vi "Calculate Tip offset.vi"() -> ()   [LabVIEW 2016]
uses:
  <vilib>/Utility/file.llb/Write Delimited Spreadsheet (DBL).vi
  Classes/Controller/Motion/Motion.lvclass
  Classes/Controller/Controller.lvclass
panel:
  in  "stop":bool
  out "XYZTheta Out":dbl[](array[numeric])
  in  "Tab Control":enum32{"Page 1", "Page 2"}(tab)
  in  "Joystick P1,P2":bool
  out "Tip Offset (XY=P1-P2)":dbl[](array[numeric]) format="%#_8g"
  in  "Write Tip Offset":bool
  out "Tip Offset (file)":dbl[](array[numeric]) format="%#_8g"
  in  "get p 2":bool
  in  "get p 1":bool
  out "P1 - P2":dbl[](array[numeric])
  out "P2":dbl[](array[numeric])
  out "P1":dbl[](array[numeric])
  out "Joystick P":dbl[](array[numeric])
  in  "Joystick":bool
  in  "needle position":dbl[](array[numeric])=[115.0, 812.0, 61.0, 0.0]
  in  "Go to needle position":bool
  # "step1"
  # "step2"
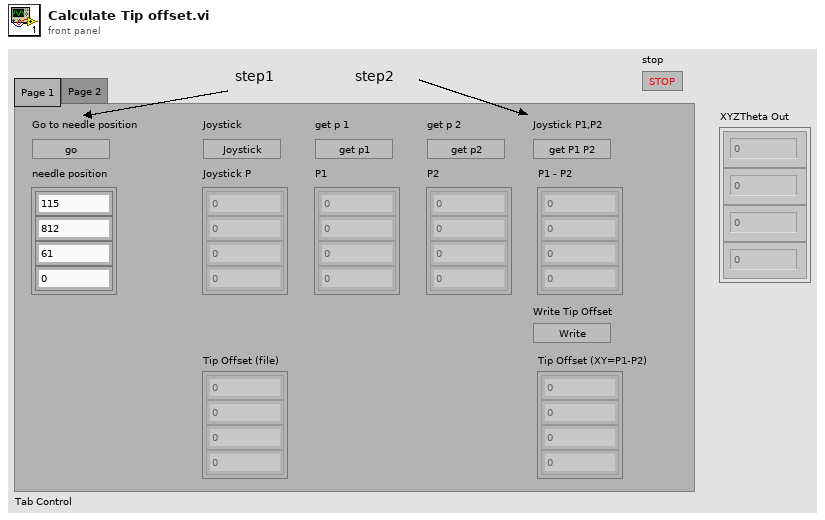
[diagram p1: front panel]
types:
  T1 = cluster{"Joystick P":refnum<vi>, "P1":refnum<vi>, "P2":refnum<vi>, "P1 - P2":refnum<vi>, "Tip Offset (file)":refnum<vi>, "Tip Offset (XY=P1-P2)":refnum<vi>}
  T2 = typedef "File Paths.ctl" = cluster{"Glue Pattern Folder":path, "Carrier Tray Folder":path, "Pick Up Tool Fixture Folder":path, "Components Folder":path, "Bellows Tool Offset.txt":path, "Pick Up Tool Offset.txt":path, "Dispense Tip Offset.txt":path, "Log Files":path}
  T3 = typedef "Controller.lvclass/Controllers.ctl" = cluster{"I-O.lvclass":refnum<class "I-O.lvclass">, "Motion.lvclass":refnum<class "Motion.lvclass">, "Dispenser.lvclass":refnum<class "Dispenser.lvclass">}
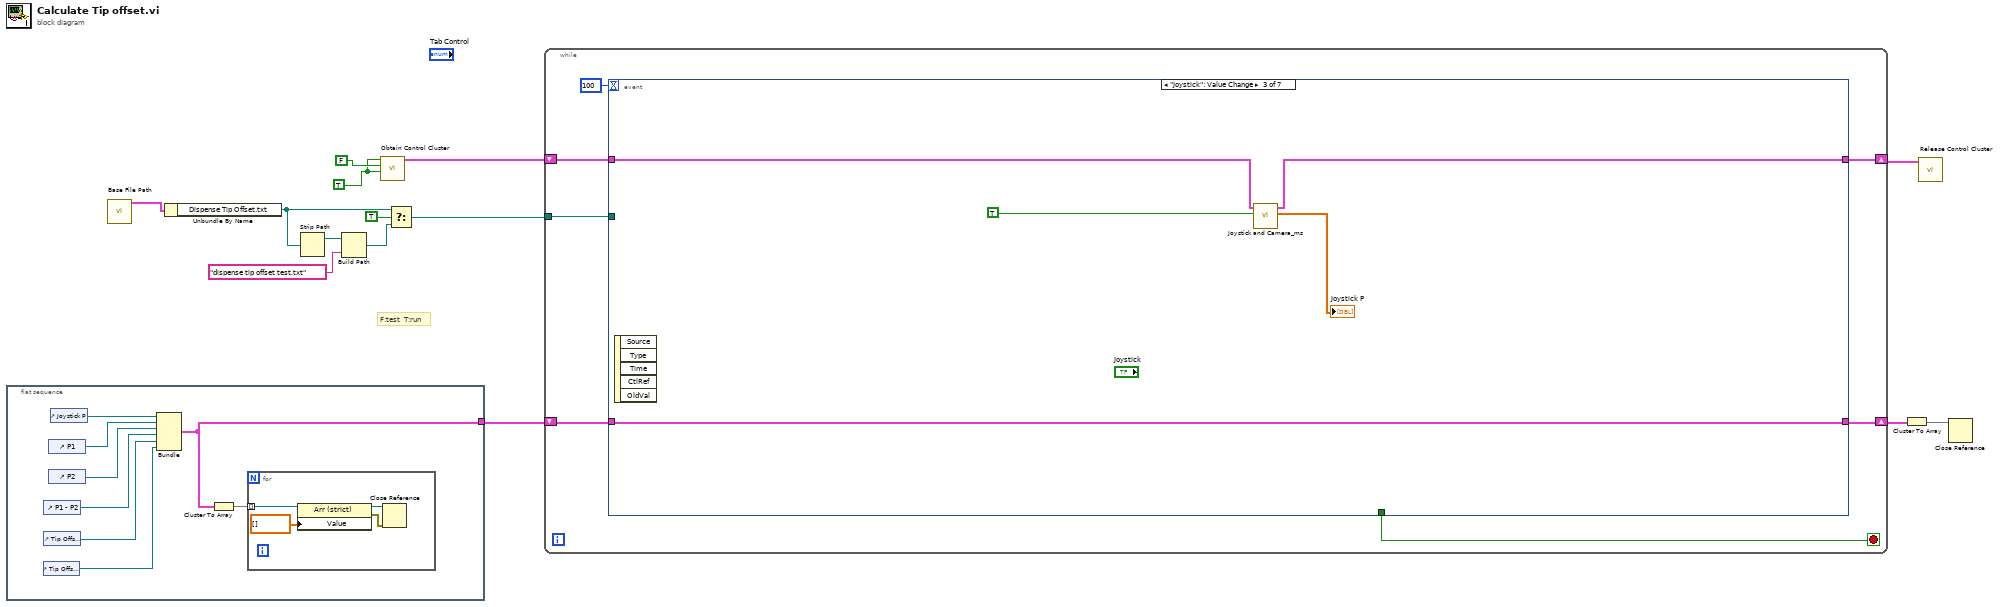
[diagram p0: block diagram]
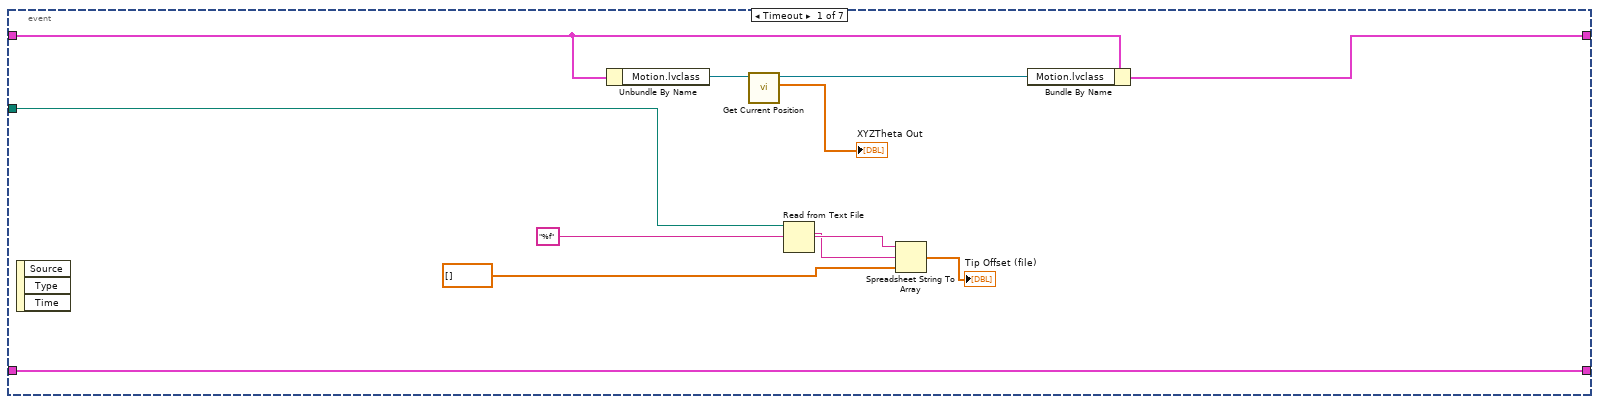
[diagram p2: hidden frame]
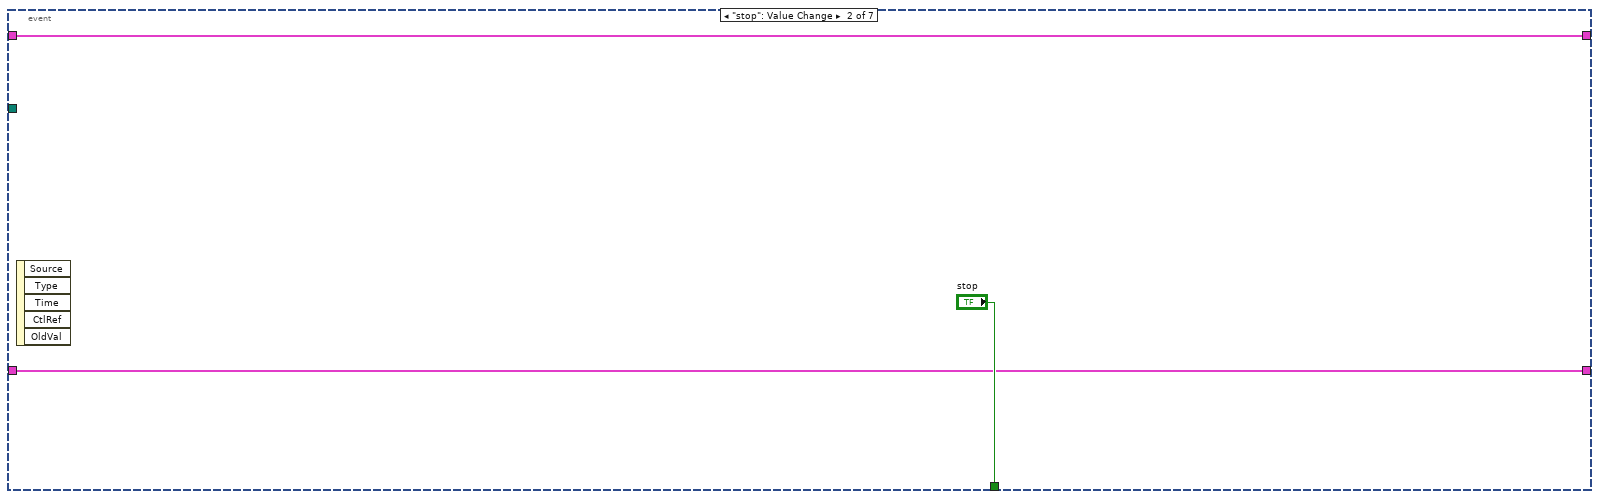
[diagram p3: hidden frame]
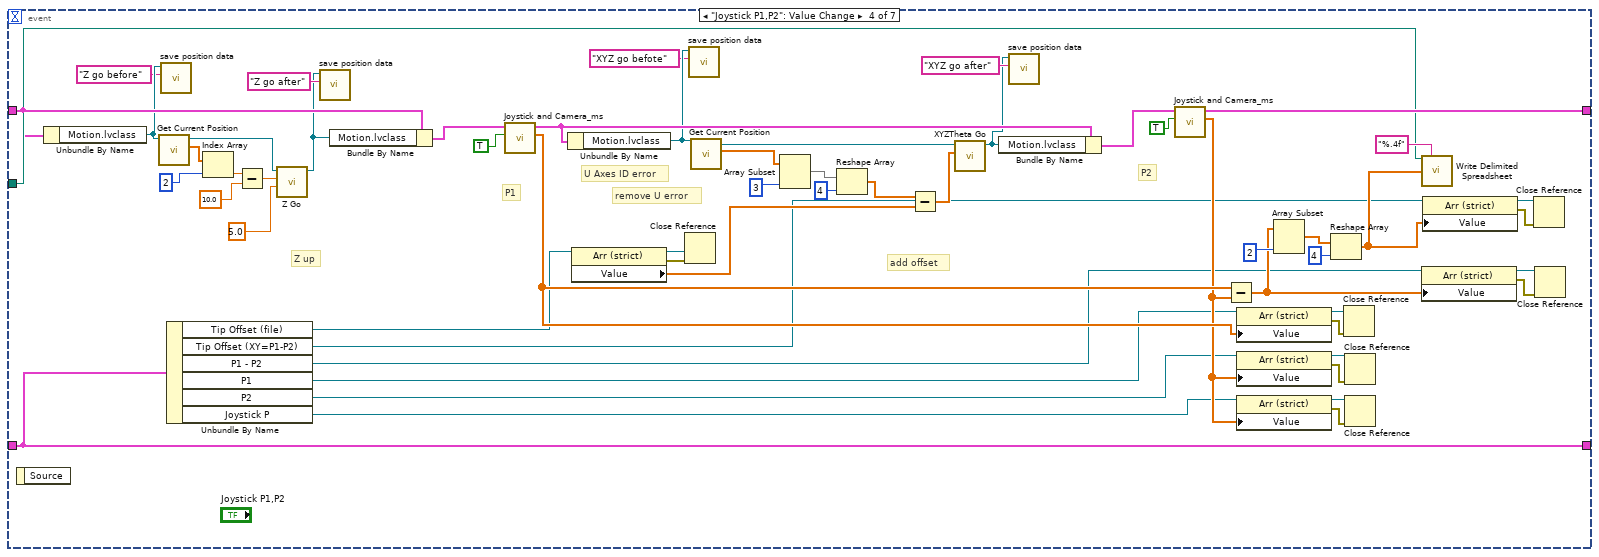
[diagram p4: hidden frame]
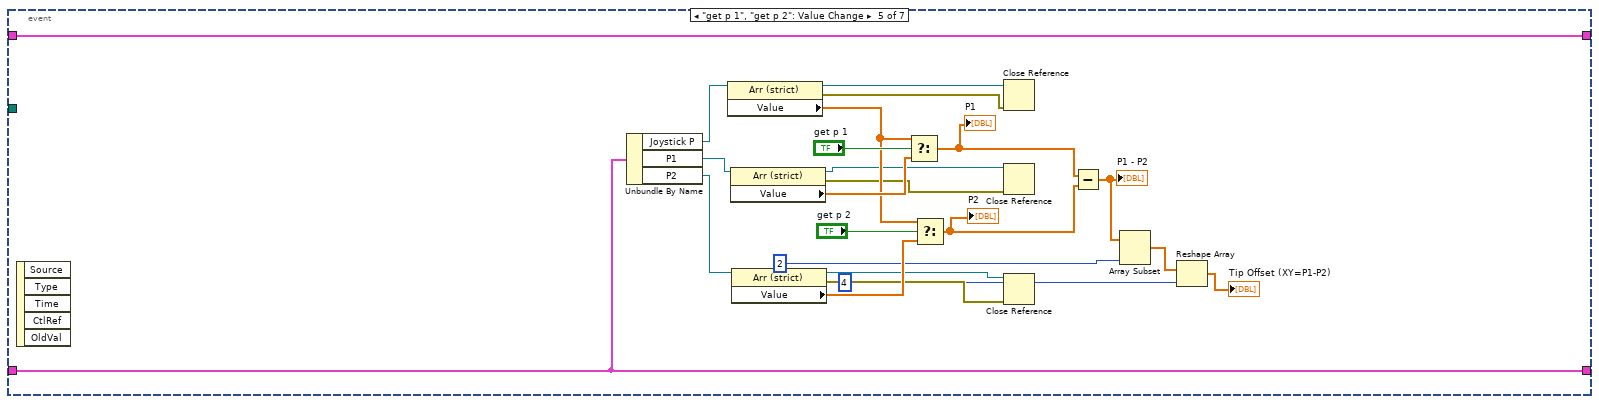
[diagram p5: hidden frame]
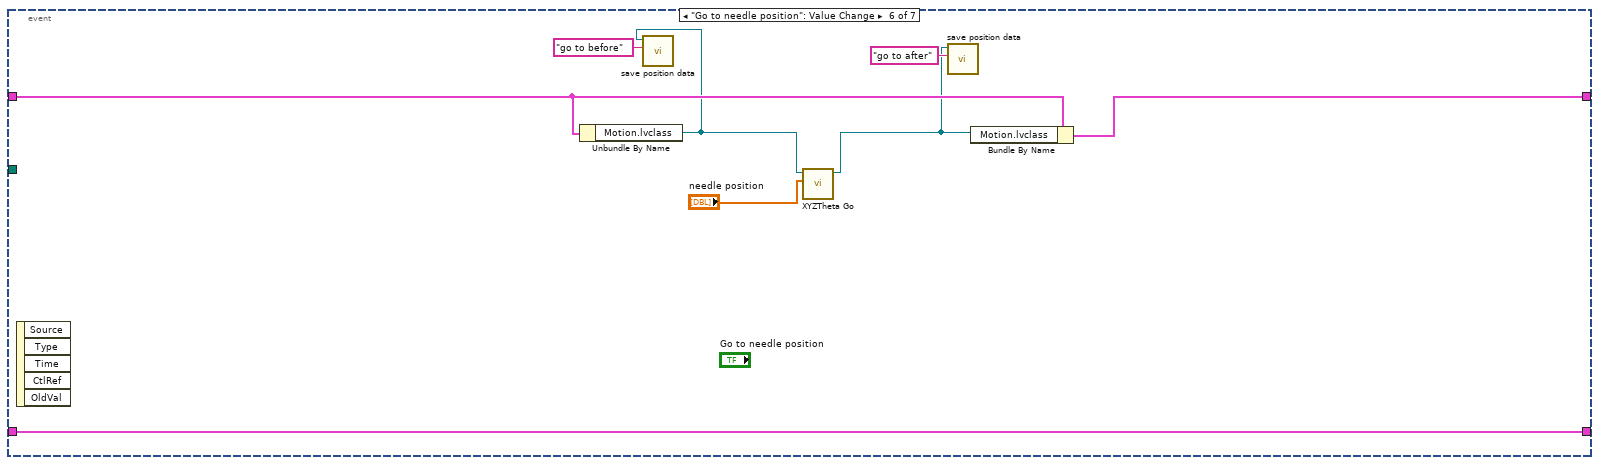
[diagram p6: hidden frame]
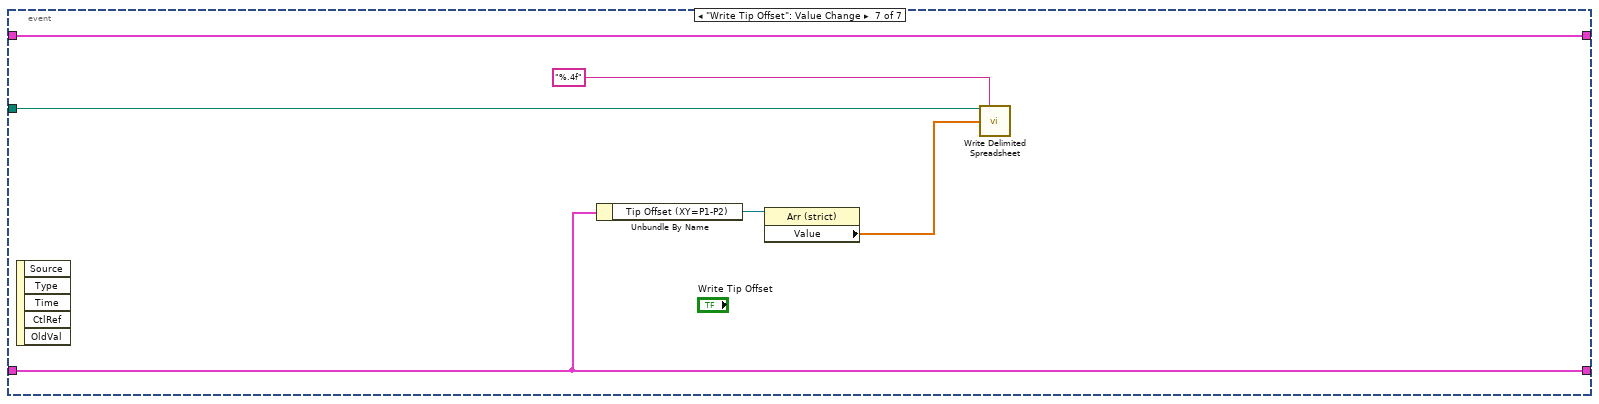
[diagram p7: hidden frame]
diagram:
  w13 = TRUE ("I/O")
  # "F:test  T:run"
  n1 = flat-sequence {
    tunnel: [w18] -> w10
    frame #0 {
      n2 = control-ref of="Tip Offset (XY=P1-P2)"() -> (w15:refnum<vi>)
      n3 = control-ref of="P1 - P2"() -> (w17:refnum<vi>)
      n4 = control-ref of="Tip Offset (file)"() -> (w16:refnum<vi>)
      n5 = control-ref of="P1"() -> (w21:refnum<vi>)
      n6 = control-ref of="P2"() -> (w20:refnum<vi>)
      n7 = control-ref of="Joystick P"() -> (w22:refnum<vi>)
      n8 = Bundle("Joystick P"=w22, "P1"=w21, "P2"=w20, "P1 - P2"=w17, "Tip Offset (file)"=w16, "Tip Offset (XY=P1-P2)"=w15) -> (w18:T1)  [unwired: 1 in]
      n9 = Cluster To Array(cluster=w18) -> (array=w19:refnum<vi>[])
      n10 = for {
        tunnel: w19 -> [w25] mode=indexing
        n11 = property class="Arr (strict)"(reference=w25, "Value"=dbl[] []) -> (reference out=w23:refnum<vi>, error out=w24:errorcluster)  [unwired: 1 in]
        n12 = Close Reference(reference=w23, error in (no error)=w24) -> ()  [unwired: 1 out]
      }
    }
  }
  n13 = call "Base File Path.vi"() -> ("Paths Out"=w4:T2)  [unwired: 11 in]
  n14 = Unbundle By Name(w4) -> ("Dispense Tip Offset.txt"=w6:path)
  n15 = Strip Path(path=w6) -> (stripped path=w8:path)  [unwired: 1 out]
  n16 = Build Path(base path=w8, name or relative path="dispense tip offset test.txt") -> (appended path=w7:path)
  n17 = call "Obtain Control Cluster.vi"("I/O"=w13, "Dispense"=FALSE, "Motion"=w13) -> ("Control Out"=w12:T3)  [unwired: 8 in]
  n18 = Select(t=w6, s=TRUE, f=w7) -> (s? t:f=w3:path)
  n19 = while {
    shift-right: [w31] -> w11
    shift-left: w12 -> [w32]
    tunnel: w3 -> [w28]
    shift-right: [w27] -> w2
    shift-left: w10 -> [w29]
    stop <- w30 stop-if-true
    n20 = event shown="[2] \"Joystick\": Value Change" {
      selector: _ -> [_ _ _ _ _ _ _]
      dyn-events: _ -> [_ _ _ _ _ _ _]
      timeout: 100 -> [_ _ _ _ _ _ _]
      tunnel: w32 -> [w42 w47 w51 w62 w133 w141 w147]
      tunnel: [w41 w47 w50 w110 w133 w140 w147] -> w31
      tunnel: [_ "stop" _ _ _ _ _] -> w30
      tunnel: w29 -> [w34 w45 w48 w98 w111 w138 w146]
      tunnel: w28 -> [w36 _ _ w75 _ _ w142]
      tunnel: [w34 w45 w48 w98 w111 w138 w146] -> w27
      event Timeout {
        n21 = event-data() -> ()  [unwired: 1 in, 3 out]
        n22 = Unbundle By Name(w42) -> ("Motion.lvclass"=w44:refnum<class "Motion.lvclass">)
        n23 = call-dynamic "Get Current Position.vi"("Motion in"=w44) -> ("XYZTheta Out"=→"XYZTheta Out":dbl[], "Motion out"=w40:refnum<class "Motion.lvclass">)  [unwired: 8 in, 1 out]
        n24 = Read from Text File(file (use dialog)=w36) -> (text=w38:string)  [unwired: 3 in, 3 out]
        n25 = Spreadsheet String To Array(format string="%f", spreadsheet string=w38, array type (2D Dbl)=dbl[] []) -> (array=→"Tip Offset (file)":dbl[])  [unwired: 1 in]
        n26 = Bundle By Name(cluster=w42, "Motion.lvclass"=w40) -> (w41:T3)
      }
      event "stop": Value Change {
        n27 = event-data() -> ()  [unwired: 1 in, 5 out]
      }
      event "Joystick": Value Change {
        n28 = event-data() -> ()  [unwired: 1 in, 5 out]
        n29 = call "Joystick and Camera_ms.vi"("VI"=TRUE, "control input"=w51) -> ("Gantry"=→"Joystick P":dbl[], "control output"=w50:T3)  [unwired: 8 in]
      }
      event "Joystick P1,P2": Value Change {
        # "Z up"
        # "P2"
        # "P1"
        # "U Axes ID error"
        # "remove U error"
        # "add offset"
        n30 = event-data() -> ()  [unwired: 1 in, 1 out]
        n31 = Unbundle By Name(w62) -> ("Motion.lvclass"=w59:refnum<class "Motion.lvclass">)
        n32 = call-dynamic "Get Current Position.vi"("Motion in"=w59) -> ("XYZTheta Out"=w69:dbl[], "Motion out"=w63:refnum<class "Motion.lvclass">)  [unwired: 8 in, 1 out]
        n33 = call "save position data.vi"("step name"="Z go before", "Motion.lvclass"=w59) -> ()  [unwired: 9 in, 1 out]
        n34 = Unbundle By Name(w98) -> ("Tip Offset (file)"=w76:refnum<vi>, "Tip Offset (XY=P1-P2)"=w77:refnum<vi>, "P1 - P2"=w80:refnum<vi>, "P1"=w81:refnum<vi>, "P2"=w82:refnum<vi>, "Joystick P"=w83:refnum<vi>)
        n35 = Index Array(array=w69, index=2) -> (element=w64:dbl)
        n36 = Subtract(x=w64, y=10.0) -> (x-y=w66:dbl)
        n37 = call-dynamic "Z Go.vi"("Speed"=5.0, "Position"=w66, "Motion in"=w63) -> ("Motion out"=w56:refnum<class "Motion.lvclass">)  [unwired: 7 in, 1 out]
        n38 = call "save position data.vi"("step name"="Z go after", "Motion.lvclass"=w56) -> ()  [unwired: 9 in, 1 out]
        n39 = Bundle By Name(cluster=w62, "Motion.lvclass"=w56) -> (w61:T3)
        n40 = call "Joystick and Camera_ms.vi"("VI"=TRUE, "control input"=w61) -> ("Gantry"=w103:dbl[], "control output"=w107:T3)  [unwired: 8 in]
        n41 = Unbundle By Name(w107) -> ("Motion.lvclass"=w60:refnum<class "Motion.lvclass">)
        n42 = property class="Arr (strict)"(reference=w76) -> (reference out=w94:refnum<vi>, error out=w95:errorcluster, "Value"=w105:dbl[])  [unwired: 1 in]
        n43 = Close Reference(reference=w94, error in (no error)=w95) -> ()  [unwired: 1 out]
        n44 = call "save position data.vi"("step name"="XYZ go befote", "Motion.lvclass"=w60) -> ()  [unwired: 9 in, 1 out]
        n45 = call-dynamic "Get Current Position.vi"("Motion in"=w60) -> ("XYZTheta Out"=w71:dbl[], "Motion out"=w106:refnum<class "Motion.lvclass">)  [unwired: 8 in, 1 out]
        n46 = Array Subset "Array Subset"(array=w71, length=3) -> (w73:dbl[])  [unwired: 1 in]
        n47 = Reshape Array "Reshape Array"(w73, 4 ("dimension size")) -> (w70:dbl[])
        n48 = Subtract(x=w70, y=w105) -> (x-y=w104:dbl[])
        n49 = call "XYZTheta Go.vi"("XYZTheta In"=w104, "Motion in"=w106) -> ("Motion out"=w53:refnum<class "Motion.lvclass">)  [unwired: 7 in, 2 out]
        n50 = Bundle By Name(cluster=w107, "Motion.lvclass"=w53) -> (w102:T3)
        n51 = call "save position data.vi"("step name"="XYZ go after", "Motion.lvclass"=w53) -> ()  [unwired: 9 in, 1 out]
        n52 = call "Joystick and Camera_ms.vi"("VI"=TRUE, "control input"=w102) -> ("Gantry"=w97:dbl[], "control output"=w110:T3)  [unwired: 8 in]
        n53 = Subtract(x=w103, y=w97) -> (x-y=w96:dbl[])
        n54 = property class="Arr (strict)"(reference=w81, "Value"=w103) -> (reference out=w92:refnum<vi>, error out=w93:errorcluster)  [unwired: 1 in]
        n55 = property class="Arr (strict)"(reference=w82, "Value"=w97) -> (reference out=w90:refnum<vi>, error out=w91:errorcluster)  [unwired: 1 in]
        n56 = property class="Arr (strict)"(reference=w83, "Value"=w97) -> (reference out=w88:refnum<vi>, error out=w89:errorcluster)  [unwired: 1 in]
        n57 = Array Subset "Array Subset"(array=w96, length=2) -> (w100:dbl[])  [unwired: 1 in]
        n58 = Reshape Array "Reshape Array"(w100, 4 ("dimension size")) -> (w78:dbl[])
        n59 = Close Reference(reference=w92, error in (no error)=w93) -> ()  [unwired: 1 out]
        n60 = Close Reference(reference=w90, error in (no error)=w91) -> ()  [unwired: 1 out]
        n61 = Close Reference(reference=w88, error in (no error)=w89) -> ()  [unwired: 1 out]
        n62 = call-poly <vilib>:"Write Delimited Spreadsheet.vi"("file path (dialog if empty)"=w75, "format (%.3f)"="%.4f", "1D data"=w78) -> ()  [unwired: 11 in, 2 out]
        n63 = property class="Arr (strict)"(reference=w80, "Value"=w96) -> (reference out=w86:refnum<vi>, error out=w87:errorcluster)  [unwired: 1 in]
        n64 = property class="Arr (strict)"(reference=w77, "Value"=w78) -> (reference out=w84:refnum<vi>, error out=w85:errorcluster)  [unwired: 1 in]
        n65 = Close Reference(reference=w84, error in (no error)=w85) -> ()  [unwired: 1 out]
        n66 = Close Reference(reference=w86, error in (no error)=w87) -> ()  [unwired: 1 out]
      }
      event "get p 1", "get p 2": Value Change {
        n67 = event-data() -> ()  [unwired: 1 in, 5 out]
        n68 = Unbundle By Name(w111) -> ("Joystick P"=w131:refnum<vi>, "P1"=w129:refnum<vi>, "P2"=w128:refnum<vi>)
        n69 = property class="Arr (strict)"(reference=w131) -> (reference out=w132:refnum<vi>, error out=w130:errorcluster, "Value"=w123:dbl[])  [unwired: 1 in]
        n70 = property class="Arr (strict)"(reference=w129) -> (reference out=w120:refnum<vi>, error out=w119:errorcluster, "Value"=w124:dbl[])  [unwired: 1 in]
        n71 = property class="Arr (strict)"(reference=w128) -> (reference out=w122:refnum<vi>, error out=w121:errorcluster, "Value"=w125:dbl[])  [unwired: 1 in]
        n72 = Select(t=w123, s="get p 1", f=w124) -> (s? t:f=w118:dbl[])
        "P1" <- w118
        n73 = Select(t=w123, s="get p 2", f=w125) -> (s? t:f=w117:dbl[])
        "P2" <- w117
        n74 = Close Reference(reference=w132, error in (no error)=w130) -> ()  [unwired: 1 out]
        n75 = Close Reference(reference=w120, error in (no error)=w119) -> ()  [unwired: 1 out]
        n76 = Close Reference(reference=w122, error in (no error)=w121) -> ()  [unwired: 1 out]
        n77 = Subtract(x=w118, y=w117) -> (x-y=w114:dbl[])
        "P1 - P2" <- w114
        n78 = Array Subset "Array Subset"(array=w114, length=2) -> (w113:dbl[])  [unwired: 1 in]
        n79 = Reshape Array "Reshape Array"(w113, 4 ("dimension size")) -> (→"Tip Offset (XY=P1-P2)":dbl[])
      }
      event "Go to needle position": Value Change {
        n80 = event-data() -> ()  [unwired: 1 in, 5 out]
        n81 = Unbundle By Name(w141) -> ("Motion.lvclass"=w136:refnum<class "Motion.lvclass">)
        n82 = call "save position data.vi"("step name"="go to before", "Motion.lvclass"=w136) -> ()  [unwired: 9 in, 1 out]
        n83 = call "XYZTheta Go.vi"("XYZTheta In"="needle position", "Motion in"=w136) -> ("Motion out"=w134:refnum<class "Motion.lvclass">)  [unwired: 7 in, 2 out]
        n84 = call "save position data.vi"("step name"="go to after", "Motion.lvclass"=w134) -> ()  [unwired: 9 in, 1 out]
        n85 = Bundle By Name(cluster=w141, "Motion.lvclass"=w134) -> (w140:T3)
      }
      event "Write Tip Offset": Value Change {
        n86 = event-data() -> ()  [unwired: 1 in, 5 out]
        n87 = Unbundle By Name(w146) -> ("Tip Offset (XY=P1-P2)"=w145:refnum<vi>)
        n88 = property class="Arr (strict)"(reference=w145) -> ("Value"=w144:dbl[])  [unwired: 1 in, 2 out]
        n89 = call-poly <vilib>:"Write Delimited Spreadsheet.vi"("file path (dialog if empty)"=w142, "format (%.3f)"="%.4f", "1D data"=w144) -> ()  [unwired: 11 in, 2 out]
      }
    }
  }
  n90 = Cluster To Array(cluster=w2) -> (array=w1:refnum<vi>[])
  n91 = call "Release Control Cluster.vi"("output cluster"=w11) -> ()  [unwired: 11 in]
  n92 = Close Reference(reference=w1) -> ()  [unwired: 1 in, 1 out]
